vi "fit3.vi"(0 "image array":dbl[][](array[numeric]), 5 "estimated parameters":dbl[](array[numeric]), 7 "parameter bounds":T1={"parameter minimum"=[1.0, 0.0, 0.0, 1.0, 1.0, -180.0, 0.0], "parameter maximum"=[255.0, 640.0, 480.0, 50.0, 50.0, 180.0, 128.0]}, 11 "error in (no error)":errorcluster, 12 "disable fit":bool) -> (2 "number of function calls":i32, 3 "Fitting Time":u32, 4 "best nonlinear fit":dbl[](array[numeric]), 6 "best fit parameters":dbl[](array[numeric])=[167.14051755898402, 39.154023858146694, 9.534043979855182, 46.30966986704069, 8.376343461684309, 10.31708372536886, 0.0], 10 "residue":dbl, 15 "error out":errorcluster)   [LabVIEW 2015]
uses:
  <vilib>/Analysis/6fits.llb/Curve Fitting Criteria.ctl
  <vilib>/Analysis/baseanly.llb/Real Determinant.vi
  <vilib>/Analysis/1siggen.llb/Ramp Pattern by Samples.vi
  <vilib>/gmath/NumericalOptimization/Nonlinear Curve Fit LM bound.vi
  <vilib>/gmath/NI_Gmath.lvlib
  <vilib>/Analysis/NI_AALPro.lvlib
  <vilib>/Analysis/NI_AALBase.lvlib
panel:
  out "Time (s)\nfI chart":u32(graph)
  out "number of samples":T2
  in  "termination":cluster{"max iteration":i32, "tolerance":dbl}={"max iteration"=100, "tolerance"=1e-06}
  # "max Amplitude"
  # "Amplitude"
  # "x max"
  # "m1 (Mean 1)"
  # "y max"
  # "m2 (Mean 2)"
  # "Width 1"
  # "wx Estimated"
  # "wy Estimated"
  # "Width 2"
  # "alpha"
  # "PI (/2)"
  # "Offset"
  # "(0) Amplitude\n(1) X-Pos\n(2) Y-Pos\n(3) width A\n(4) Width B\n(5) angle (DEG)\n(6) Offset"
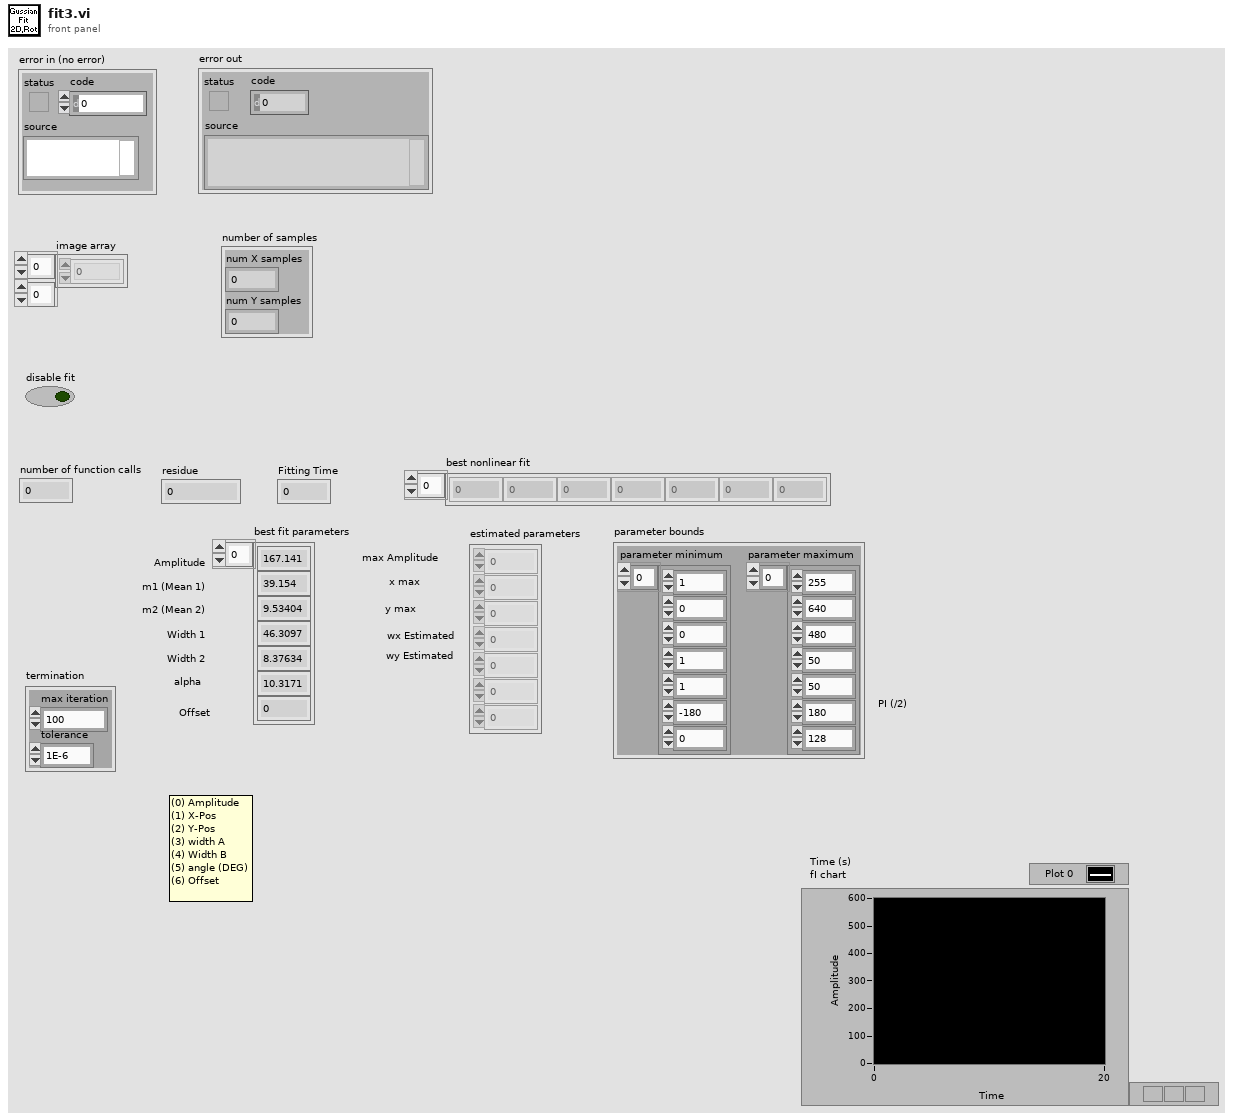
[diagram p1: front panel]
types:
  T1 = cluster{"parameter minimum":dbl[], "parameter maximum":dbl[]}
  T2 = cluster{"num X samples":i32, "num Y samples":i32}
  T3 = typedef "NI_AALPro.lvlib/Curve Fitting Criteria.ctl" = u16
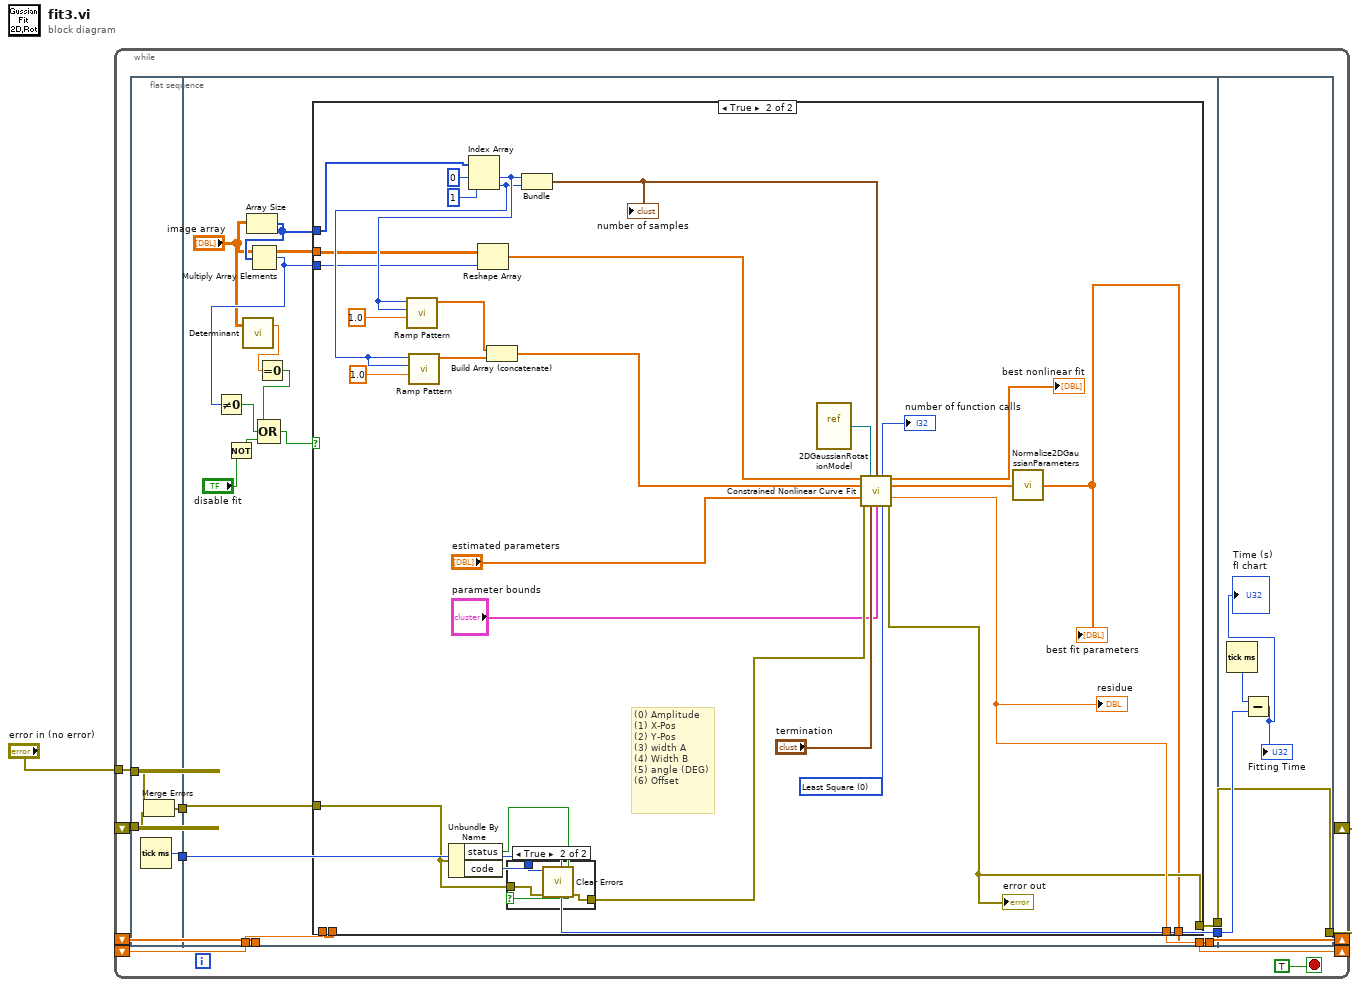
[diagram p0: block diagram]
diagram:
  n1 = while {
    shift-right: [w10] -> _
    shift-left: _ -> [w9]
    shift-right: [w8] -> _
    shift-left: _ -> [w7]
    shift-right: [w6] -> _
    shift-left: _ -> [w4]
    tunnel: "error in (no error)" -> [w2]
    stop <- TRUE stop-if-true
    n2 = flat-sequence {
      tunnel: [w17] -> w13
      tunnel: w4 -> [w16]
      tunnel: [w14] -> w3
      tunnel: w2 -> [w15]
      tunnel: w13 -> [w33]
      tunnel: [w33] -> w12
      tunnel: [w31] -> w10
      tunnel: w9 -> [w18]
      tunnel: [w32] -> w8
      tunnel: w7 -> [w19]
      tunnel: [w30] -> w5
      tunnel: w3 -> [w29]
      tunnel: w12 -> [w72]
      tunnel: [w71] -> w6
      tunnel: w5 -> [w71]
      frame #0 {
        n3 = Tick Count (ms)() -> (millisecond timer value=w17:u32)
        n4 = Merge Errors(w15, w16) -> (w14:errorcluster)
      }
      frame #1 {
        n5 = Not(x="disable fit") -> (.not. x?=w23:bool)
        n6 = call-poly <vilib>:"Determinant.vi"("Input Matrix"="image array") -> ("determinant"=w21:dbl)  [unwired: 1 in, 1 out]
        n7 = Array Size(array="image array") -> (size(s)=w25:i32[])
        n8 = Multiply Array Elements(1:w25) -> (0:w24:i32)
        n9 = Not Equal To 0?(x=w24) -> (x != 0?=w28:bool)
        n10 = Equal To 0?(x=w21) -> (x = 0?=w20:bool)
        n11 = Compound Arithmetic op=OR(w20, w28, w23) -> (w26:bool)
        n12 = case shown="True" w26 {
          tunnel: w25 -> [_ w56]
          tunnel: [w34 w51] -> w32
          tunnel: [w35 w42] -> w31
          tunnel: "image array" -> [_ w41]
          tunnel: [w36 w50] -> w30
          tunnel: w29 -> [w36 w47]
          tunnel: w24 -> [_ w45]
          tunnel: w19 -> [w34 _]
          tunnel: w18 -> [w35 _]
          frame False {
          }
          frame True {
            w58 = T3 0 items=["Least Square", "Least Absolute Residual", "Bisquare"] ("method")
            # "(0) Amplitude\n(1) X-Pos\n(2) Y-Pos\n(3) width A\n(4) Width B\n(5) angle (DEG)\n(6) Offset"
            n13 = Unbundle By Name(w47) -> ("status"=w49:bool, "code"=w48:i32)
            n14 = Index Array(array=w56, index #1=0 ("index"), index #2=1 ("index")) -> (element #1=w53:i32, element #2=w52:i32)
            n15 = call-poly <vilib>:"Ramp Pattern.vi"("start"=1.0, "end"=w53, "samples"=w53) -> ("Ramp Pattern"=w65:dbl[])  [unwired: 7 in, 1 out]
            n16 = call-poly <vilib>:"Ramp Pattern.vi"("start"=1.0, "end"=w52, "samples"=w52) -> ("Ramp Pattern"=w64:dbl[])  [unwired: 7 in, 1 out]
            n17 = Reshape Array(w41, w45) -> (w40:dbl[])
            n18 = Build Array (concatenate)(w65, w64) -> (w59:dbl[])
            n19 = case shown="True" w49 {
              tunnel: w48 -> [_ w69]
              tunnel: w47 -> [w66 w68]
              tunnel: [w66 w67] -> w46
              frame False {
              }
              frame True {
                n20 = call <vilib>:"Clear Errors.vi"("error in (no error)"=w68, "specific error code to clear (0: all)"=w69) -> ("error out"=w67:errorcluster)  [unwired: 4 in, 1 out]
              }
            }
            n21 = Bundle(w53, w52) -> (w57:cluster{i32, i32})  [unwired: 1 out]
            "number of samples" <- w57
            n22 = vi-ref "2DGaussianRotationModel.vi"() -> (w37:refnum<vi>)
            n23 = call-poly <vilib>:"Constrained Nonlinear Curve Fit.vi"("Y"=w40, "f(x,a)"=w37, "data"=w57, "X"=w59, "initial parameters"="estimated parameters", "error in (no error)"=w46, "termination"="termination", "parameter bounds"="parameter bounds", "method"=w58) -> ("number of function calls"=→"number of function calls":i32, "best nonlinear fit"=→"best nonlinear fit":dbl[], "best fit parameters"=w43:dbl[], "residue"=w51:dbl, "error out"=w50:errorcluster)  [unwired: 1 in, 1 out]
            "error out" <- w50
            "residue" <- w51
            n24 = call "Normalize2DGaussianParameters.vi"("best fit parameters IN"=w43) -> ("best fit parameters OUT"=w42:dbl[])
            "best fit parameters" <- w42
          }
        }
      }
      frame #2 {
        n25 = Tick Count (ms)() -> (millisecond timer value=w73:u32)
        n26 = Subtract(x=w73, y=w72) -> (x-y=→"Fitting Time" →"Time (s)\nfI chart":u32)
      }
    }
  }
